vi "Destroy REST Client.vi"(8 "error in (no error)":errorcluster, 11 "REST Client in":refnum<class "REST Client.lvclass">) -> (0 "error out":errorcluster)   [LabVIEW 2018, in "REST Client_JKI.lvlib" / "REST Client.lvclass"]
doc: "Destroy REST client reference."
uses:
  REST Client.lvclass
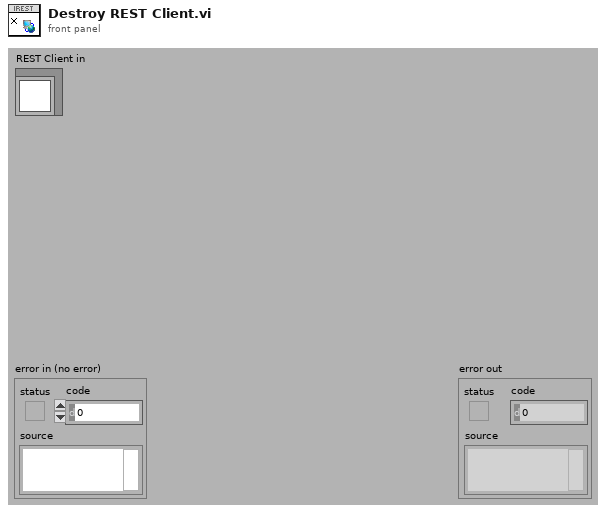
[diagram p1: front panel]
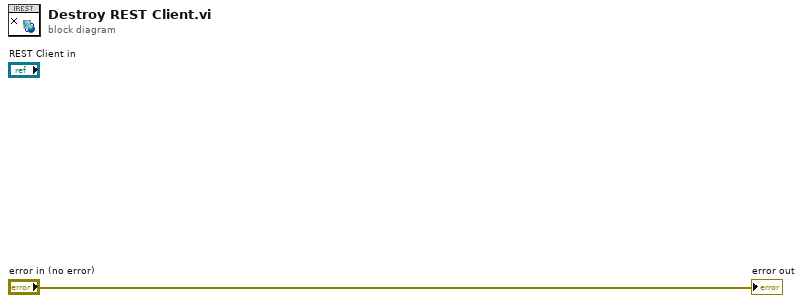
[diagram p0: block diagram]
diagram:
  "error out" <- "error in (no error)"
